vi "Send RX Message.vi"(8 "error in (no error)":errorcluster, 11 "RxTx in":refnum<class "RxTx.lvclass">) -> (0 "error out":errorcluster, 3 "RxTx out":refnum<class "RxTx.lvclass">)   [LabVIEW 2018, in "RxTx.lvclass"]
doc: "Send Rx Message"
uses:
  RxTx.lvclass
  RxTx.lvclass/RxTx.ctl
panel:
  in  "element":string
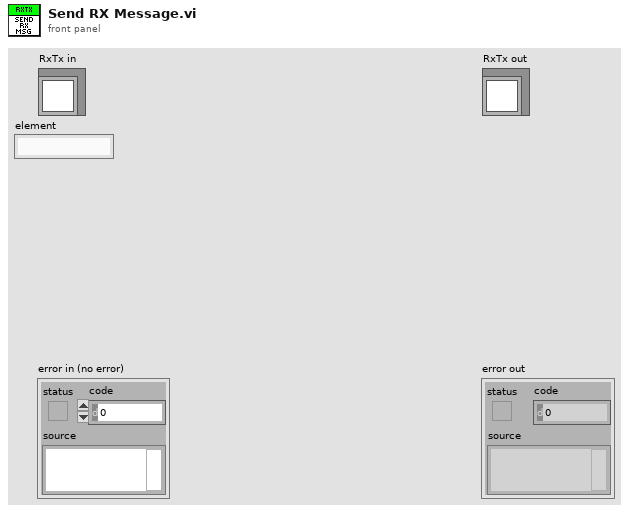
[diagram p1: front panel]
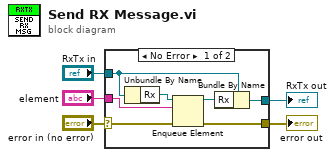
[diagram p0: block diagram]
diagram:
  n1 = case shown="No Error" "error in (no error)" {
    selector: "error in (no error)" -> [w11 w14]
    tunnel: [w12 w14] -> w3
    tunnel: [w8 w13] -> w2
    tunnel: "RxTx in" -> [w9 w13]
    tunnel: "element" -> [w6 _]
    frame No Error {
      n2 = Unbundle By Name(w9) -> ("Rx"=w10:refnum<queue>)
      n3 = Enqueue Element(queue=w10, element=w6, error in (no error)=w11) -> (queue out=w7:refnum<queue>, error out=w12:errorcluster)  [unwired: 1 in, 1 out]
      n4 = Bundle By Name(cluster=w9, "Rx"=w7) -> (w8:refnum<class "RxTx.lvclass">)
    }
    frame Error {
    }
  }
  "error out" <- w3
  "RxTx out" <- w2
